vi "Session6FFrameDLC3.vi"(8 "errin":errorcluster, 9 "Énum":enum16{"PDU", "CMOD"}(ring)=enum."CMOD", 10 "ChanelIn":T1, 11 "IDnumber":u32 format="%.0x") -> (0 "errout":errorcluster, 1 "trouvé":bool, 2 "Identique":bool, 3 "Identifier":u32 format="%x")   [LabVIEW 2020]
uses:
  PCAN Basic/Controls/Channel.ctl
  Alex_Peak_lib/PEAK_lib_ALEX.lvlib
  PCAN Basic/PCANBasic.lvlib
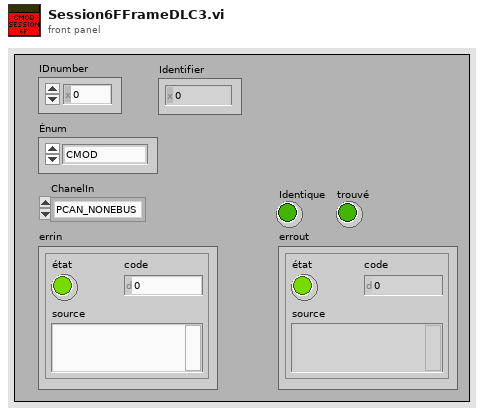
[diagram p1: front panel]
types:
  T1 = typedef "PCANBasic.lvlib/Channel.ctl" = enum16{"PCAN_NONEBUS", "not used1", "not used2", "not used3", "not used4", "not used5", "not used6", "not used7", "not used8", "not used9", "not used10", "not used11", "not used12", "not used13", "not used14", "not used15", "not used16", "not used17", "not used18", "not used19", "not used20", "not used21", "not used22", "not used23", "not used24", "not used25", "not used26", "not used27", "not used28", "not used29", "not used30", "not used31", "not used32", "PCAN_ISABUS1", "PCAN_ISABUS2", "PCAN_ISABUS3", "PCAN_ISABUS4", "PCAN_ISABUS5", "PCAN_ISABUS6", "PCAN_ISABUS7", "PCAN_ISABUS8", "not used41", "not used42", "not used43", "not used44", "not used45", "not used46", "not used47", "not used48", "PCAN_DNGBUS1", "not used50", "not used51", "not used52", "not used53", "not used54", "not used55", "not used56", "not used57", "not used58", "not used59", "not used60", "not used61", "not used62", "not used63", "not used64", "PCAN_PCIBUS1", "PCAN_PCIBUS2", "PCAN_PCIBUS3", "PCAN_PCIBUS4", "PCAN_PCIBUS5", "PCAN_PCIBUS6", "PCAN_PCIBUS7", "PCAN_PCIBUS8", "not used73", "not used74", "not used75", "not used76", "not used77", "not used78", "not used79", "not used80", "PCAN_USBBUS1", "PCAN_USBBUS2", "PCAN_USBBUS3", "PCAN_USBBUS4", "PCAN_USBBUS5", "PCAN_USBBUS6", "PCAN_USBBUS7", "PCAN_USBBUS8", "Not used89", "Not used90", "Not used91", "Not used92", "Not used93", "Not used94", "Not used95", "Not used96", "PCAN_PCCBUS1", "PCAN_PCCBUS2"}
  T2 = cluster{"ID":u32, "MSGTYPE":u8, "LEN":u8, "DATA[0]":u8, "DATA[1]":u8, "DATA[2]":u8, "DATA[3]":u8, "DATA[4]":u8, "DATA[5]":u8, "DATA[6]":u8, "DATA[7]":u8}
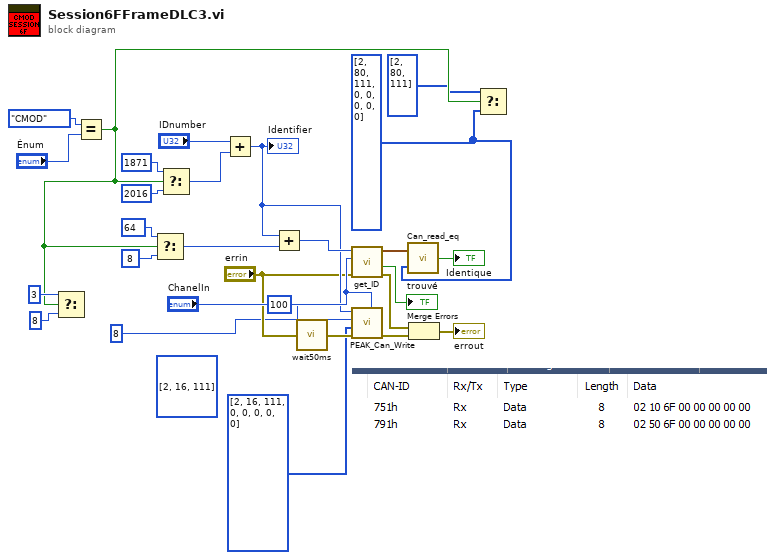
[diagram p0: block diagram]
diagram:
  (unwired) u8[] [2, 16, 111] ("CAN Data")
  w2 = u8[] [2, 80, 111, 0, 0, 0, 0, 0] ("TrameJeVeux")
  n1 = Equal?(x=enum16{"PDU", "CMOD"}."CMOD" ("Énum 2"), y="Énum") -> (x = y?=w5:bool)
  n2 = Select(t=3 ("cas vrai"), s=w5, f=8) -> ()  [unwired: 1 out]
  n3 = Select(t=u32 64 ("Identifier"), s=w5, f=u32 8 ("cas faux")) -> (s? t:f=w10:u32)
  n4 = Select(t=u32 1871 ("Identifier"), s=w5, f=u32 2016 ("cas faux")) -> (s? t:f=w14:u32)
  n5 = Add(x="IDnumber", y=w14) -> (x+y=w23:u32)
  "Identifier" <- w23
  n6 = Add(x=w23, y=w10) -> (x+y=w28:u32)
  n7 = call "wait50ms.vi"("attente (ms)"=u32 100, "errin"="errin") -> ("errout"=w21:errorcluster)  [unwired: 13 in]
  n8 = call "get_ID.vi"("errin"="errin", "ChannelIn"="ChanelIn", "Identifier"=w28) -> ("errout"=w19:errorcluster, "trouvé"=→"trouvé":bool, "Messout"=w25:T2)  [unwired: 5 in, 1 out]
  n9 = call "PEAK_Can_Write.vi"("CAN Handle"="ChanelIn", "errin"=w21, "CAN Data"=u8[] [2, 16, 111, 0, 0, 0, 0, 0], "DLC (8)"=u8 8, "Identifier"=w23) -> ("errout"=w18:errorcluster)  [unwired: 6 in]
  n10 = call "Can_read_eq.vi"("TrameJeVeux"=w2, "MessIN"=w25) -> ("Identique"=→"Identique":bool)
  n11 = Merge Errors(w19, w18) -> (→"errout":errorcluster)
  n12 = Select(t=u8[] [2, 80, 111] ("TrameJeVeux"), s=w5, f=w2) -> ()  [unwired: 1 out]
